vi "toangle.vi"(10 "Numeric":dbl format="%#_13g", 11 "number":cluster{dbl, dbl}) -> (3 "atan2(y,x)":dbl)   [LabVIEW 2015]
panel:
  out "sqrt(x)":dbl
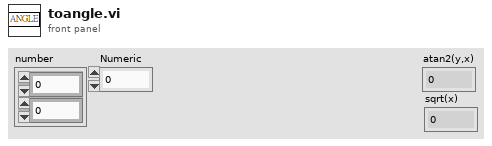
[diagram p1: front panel]
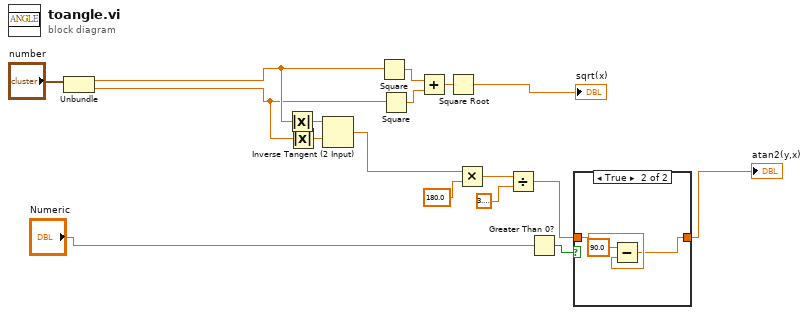
[diagram p0: block diagram]
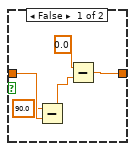
[diagram p2: hidden frame]
diagram:
  n1 = Unbundle("number") -> (w11:dbl, w10:dbl)
  n2 = Absolute Value(x=w11) -> (abs(x)=w14:dbl)
  n3 = Absolute Value(x=w10) -> (abs(x)=w13:dbl)
  n4 = Inverse Tangent (2 Input)(1:w13, 2:w14) -> (0:w6:dbl)
  n5 = Square(x=w11) -> (x^2=w17:dbl)
  n6 = Square(x=w10) -> (x^2=w16:dbl)
  n7 = Add(x=w17, y=w16) -> (x+y=w15:dbl)
  n8 = Square Root(x=w15) -> (sqrt(x)=→"sqrt(x)":dbl)
  n9 = Multiply(x=w6, y=180.0) -> (x*y=w7:dbl)
  n10 = Divide(x=w7, y=3.141592653589793) -> (x/y=w2:dbl)
  n11 = Greater Than 0?(x="Numeric") -> (x > 0?=w3:bool)
  n12 = case shown="True" w3 {
    tunnel: w2 -> [w19 w24]
    tunnel: [w21 w23] -> w1
    frame False {
      n13 = Subtract(x=90.0, y=w19) -> (x-y=w20:dbl)
      n14 = Subtract(x=0.0, y=w20) -> (x-y=w21:dbl)
    }
    frame True {
      n15 = Subtract(x=90.0, y=w24) -> (x-y=w23:dbl)
    }
  }
  "atan2(y,x)" <- w1
